vi "read_error_to_process.vi"(11 "Error in":refnum<class "Error.lvclass">) -> (2 "error_to_process":errorcluster)   [LabVIEW 2023, in "Error Handling Interface.lvlib" / "Error.lvclass"]
uses:
  Error.lvclass
  Error.lvclass/Error.ctl
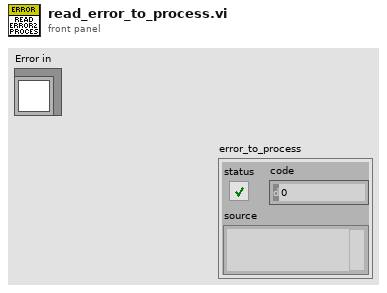
[diagram p1: front panel]
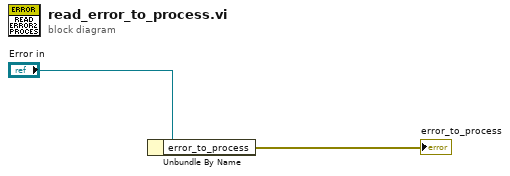
[diagram p0: block diagram]
diagram:
  n1 = Unbundle By Name("Error in") -> ("error_to_process"=→"error_to_process":errorcluster)
